vi "Rotate Face 5.vi"(10 "Pretransform Rubix Array":T1[][](array[typedef]), 11 "Command":T2=-1 items=["Up"=-1, "Down"=1]) -> (1 "Axis":cluster{"X":sgl, "Y":sgl, "Z":sgl}={"X"=1.0, "Y"=0.0, "Z"=0.0}, 2 "Transform Rubix Array":T1[][](array[typedef]), 3 "Facets to move":T1[](array[typedef]))   [LabVIEW 2019]
uses:
  Rotate array command.ctl
  Rubix Array data type.ctl
  section movement.ctl
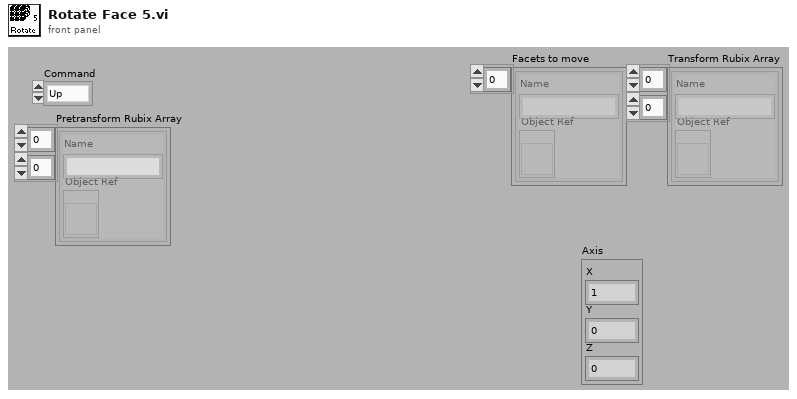
[diagram p1: front panel]
types:
  T1 = typedef "Rubix Array data type.ctl" = cluster{"Object Ref":refnum<vi>, "Name":string}
  T2 = typedef "Rotate array command.ctl" = i32
  T3 = typedef "section movement.ctl" = enum16{"Left", "Right"}
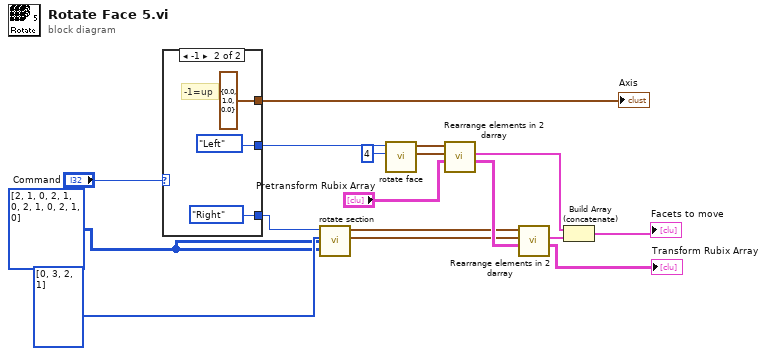
[diagram p0: block diagram]
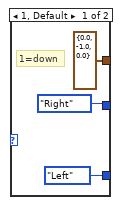
[diagram p2: hidden frame]
diagram:
  w3 = i32[][] [[2, 1, 0], [2, 1, 0], [2, 1, 0], [2, 1, 0]] ("From Facet")
  n1 = case shown="-1" "Command" {
    tunnel: [cluster{"X":sgl, "Y":sgl, "Z":sgl} {"X"=0.0, "Y"=-1.0, "Z"=0.0} ("Axis") cluster{"X":sgl, "Y":sgl, "Z":sgl} {"X"=0.0, "Y"=1.0, "Z"=0.0} ("Axis")] -> w11
    tunnel: [section_movement."Right" ("Direction") section_movement."Left" ("Direction")] -> w9
    tunnel: [section_movement."Left" ("Enum") section_movement."Right" ("Enum")] -> w7
    frame 1, Default {
      # "1=down"
    }
    frame -1 {
      # "-1=up"
    }
  }
  "Axis" <- w11
  n2 = call "rotate section.vi"("To Facet"=w3, "From Facet"=w3, "From"=i32[] [0, 3, 2, 1] ("From 2"), "Enum"=w7) -> ("To"=w5:cluster{"row":i32, "column":i32}[], "From"=w6:cluster{"row":i32, "column":i32}[])  [unwired: 6 in]
  n3 = call "rotate face.vi"("Face to act on"=4, "Direction"=w9) -> ("To"=w15:cluster{"row":i32, "column":i32}[], "From"=w16:cluster{"row":i32, "column":i32}[])  [unwired: 8 in]
  n4 = call "Rearrange elements in 2 darray.vi"("Pretransform Rubix Array"="Pretransform Rubix Array", "To"=w15, "From"=w16) -> ("Transform Rubix Array"=w12:T1[][], "Facets to move"=w17:T1[])  [unwired: 7 in]
  n5 = call "Rearrange elements in 2 darray.vi"("Pretransform Rubix Array"=w12, "To"=w5, "From"=w6) -> ("Transform Rubix Array"=→"Transform Rubix Array":T1[][], "Facets to move"=w14:T1[])  [unwired: 7 in]
  n6 = Build Array (concatenate)(w17, w14) -> (→"Facets to move":T1[])
